vi "InitialConditions FGV.vi"(8 "error in (no error)":errorcluster, 9 "Y0":dbl, 10 "X0":dbl, 11 "Enum":T1) -> (0 "error out":errorcluster, 1 "y0":dbl, 2 "x0":dbl)   [LabVIEW 2017, in "admittanceControllerLibrary.lvlib"]
doc: "This FGV contains the starting x and y positions for each reaching movement, required for the minimum jerk trajectory."
uses:
  admittanceControllerLibrary.lvlib
  Controls/initial conditions control.ctl
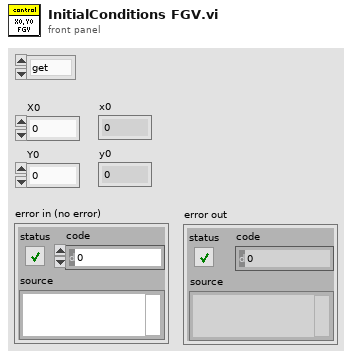
[diagram p1: front panel]
types:
  T1 = typedef "admittanceControllerLibrary.lvlib/initial conditions control.ctl" = enum16{"get", "set"}
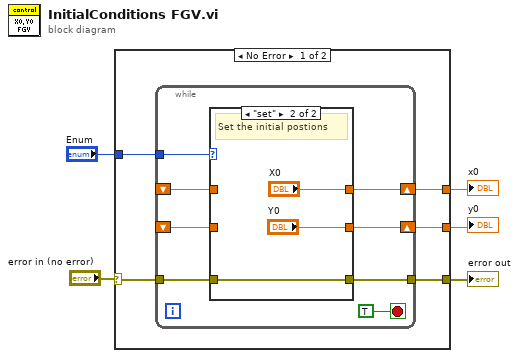
[diagram p0: block diagram]
diagram:
  n1 = case shown="No Error" "error in (no error)" {
    selector: "error in (no error)" -> [w7 w25]
    tunnel: "Enum" -> [w10 _]
    tunnel: [w9 _] -> w4
    tunnel: [w8 _] -> w3
    tunnel: [w6 w25] -> w1
    frame No Error {
      n2 = while {
        shift-right: [w13] -> w9
        shift-left: _ -> [w16]
        shift-right: [w14] -> w8
        shift-left: _ -> [w15]
        tunnel: w10 -> [w17]
        tunnel: w7 -> [w12]
        tunnel: [w11] -> w6
        stop <- TRUE stop-if-true
        n3 = case shown="\"set\"" w17 {
          tunnel: [w21 "X0"] -> w13
          tunnel: [w20 "Y0"] -> w14
          tunnel: w16 -> [w21 _]
          tunnel: w15 -> [w20 _]
          tunnel: w12 -> [w19 w22]
          tunnel: [w19 w22] -> w11
          frame "get", Default {
            # "Get the initial positions"
          }
          frame "set" {
            # "Set the initial postions"
          }
        }
      }
    }
    frame Error {
    }
  }
  "error out" <- w1
  "x0" <- w4
  "y0" <- w3
